vi "Add Lookup Event Listener.vi"(6 "Base Class (LabVIEW Object)":refnum<class>, 8 "error in (no error)":errorcluster, 9 "Lookup Listener User Event":refnum<user-event>, 11 "Lookup Service in":refnum<data-value>) -> (0 "error out":errorcluster, 3 "Lookup Service out":refnum<data-value>)   [LabVIEW 2014, in "LVCOOOP.lvlib" / "Lookup API.lvlib" / "Lookup Service.lvclass"]
doc: "Add a user-event listener to the Lookup. The user event will be triggered if the contents of the lookup for the specified class change."
uses:
  Lookup Service.lvclass
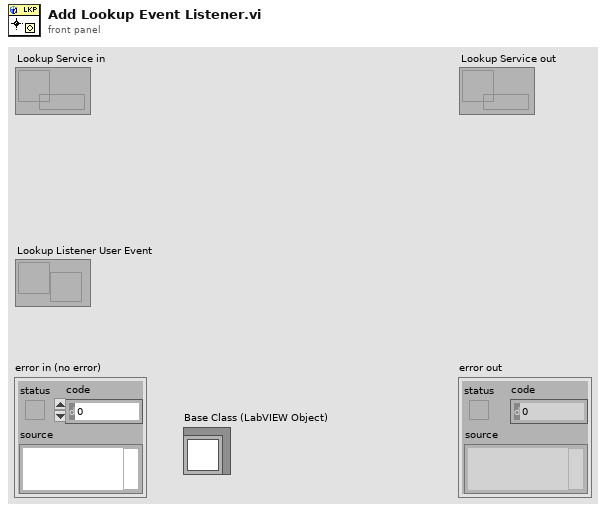
[diagram p1: front panel]
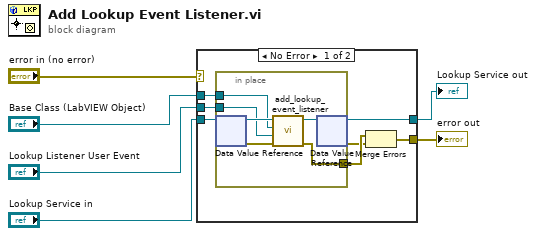
[diagram p0: block diagram]
diagram:
  n1 = case shown="No Error" "error in (no error)" {
    selector: "error in (no error)" -> [_ w21]
    tunnel: "Lookup Service in" -> [w13 w20]
    tunnel: [w12 w20] -> w4
    tunnel: "Base Class (LabVIEW Object)" -> [w11 _]
    tunnel: "Lookup Listener User Event" -> [w10 _]
    tunnel: [w7 w21] -> w1
    frame No Error {
      n2 = in-place {
        in-place-border: w11 -> [w18]
        in-place-border: w10 -> [w17]
        in-place-border: [w15] -> w9
        n3 = in-place-dvr #1(w13) -> (w19:refnum<class "Lookup Service.lvclass">, w16:errorcluster)
        n4 = call-dynamic "add_lookup_event_listener.vi"("error in (no error)"=w16, "Lookup Listener User Event"=w17, "Base Class (LabVIEW Object)"=w18, "Lookup Service in"=w19) -> ("error out"=w15:errorcluster, "Lookup Service out"=w14:refnum<class "Lookup Service.lvclass">)  [unwired: 6 in]
        n5 = in-place-dvr #1(w14) -> (w12:refnum<data-value>, w8:errorcluster)
      }
      n6 = Merge Errors(w9, w8) -> (w7:errorcluster)
    }
    frame Error {
    }
  }
  "error out" <- w1
  "Lookup Service out" <- w4
